vi "Initiate FGEN Generation and Scope Acquisition.vi"(8 "error in (no error)":errorcluster, 10 "FGEN Resources in":refnum<k15>[](array[refnum]), 11 "Scope Resources in":refnum<k15>[](array[refnum])) -> (0 "error out":errorcluster, 2 "FGEN Resources out":refnum<k15>[](array[refnum]), 3 "Scope Resources out":refnum<k15>[](array[refnum]))   [LabVIEW 2024]
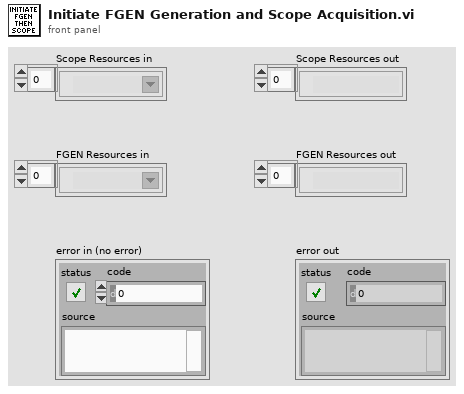
[diagram p1: front panel]
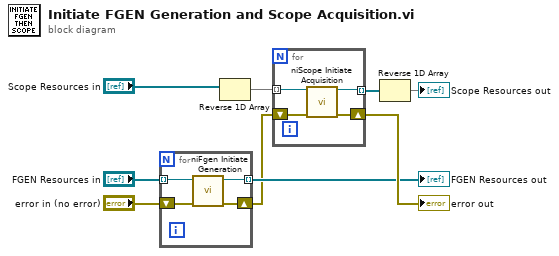
[diagram p0: block diagram]
diagram:
  n1 = for {
    tunnel: "FGEN Resources in" -> [w13] mode=indexing
    shift-right: [w11] -> w6
    shift-left: "error in (no error)" -> [w12]
    tunnel: [w10] -> w7 mode=indexing
    n2 = call <instrlib>:"niFgen Initiate Generation.vi"("error in (no error)"=w12, "Instrument Handle"=w13) -> ("error out"=w11:errorcluster, "Instrument Handle Out"=w10:refnum<k15>)  [unwired: 8 in]
  }
  "FGEN Resources out" <- w7
  n3 = Reverse 1D Array(array="Scope Resources in") -> (reversed array=w2:refnum<k15>[])
  n4 = for {
    tunnel: w2 -> [w17] mode=indexing
    tunnel: [w16] -> w3 mode=indexing
    shift-right: [w14] -> w8
    shift-left: w6 -> [w15]
    n5 = call <instrlib>:"niScope Initiate Acquisition.vi"("instrument handle"=w17, "error in"=w15) -> ("instrument handle out"=w16:refnum<k15>, "error out"=w14:errorcluster)  [unwired: 12 in]
  }
  "error out" <- w8
  n6 = Reverse 1D Array(array=w3) -> (reversed array=→"Scope Resources out":refnum<k15>[])
